vi "Terminate Condition Extract Time.vi"(8 "error in":errorcluster, 11 "Normalized Timer Array in":dbl[][](array[numeric])) -> (0 "error out":errorcluster, 3 "Condition (b) Equilibrium?":bool)   [LabVIEW 2023]
panel:
  out "Numeric":i32
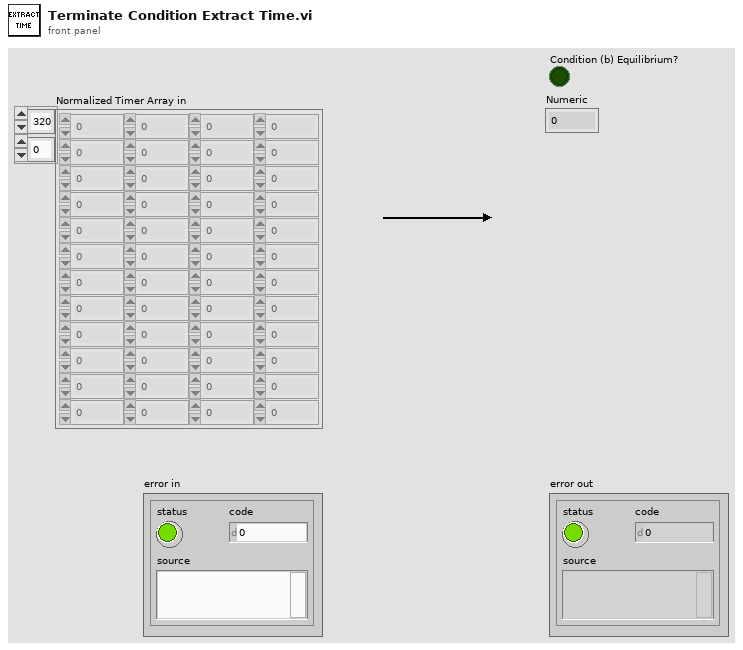
[diagram p1: front panel]
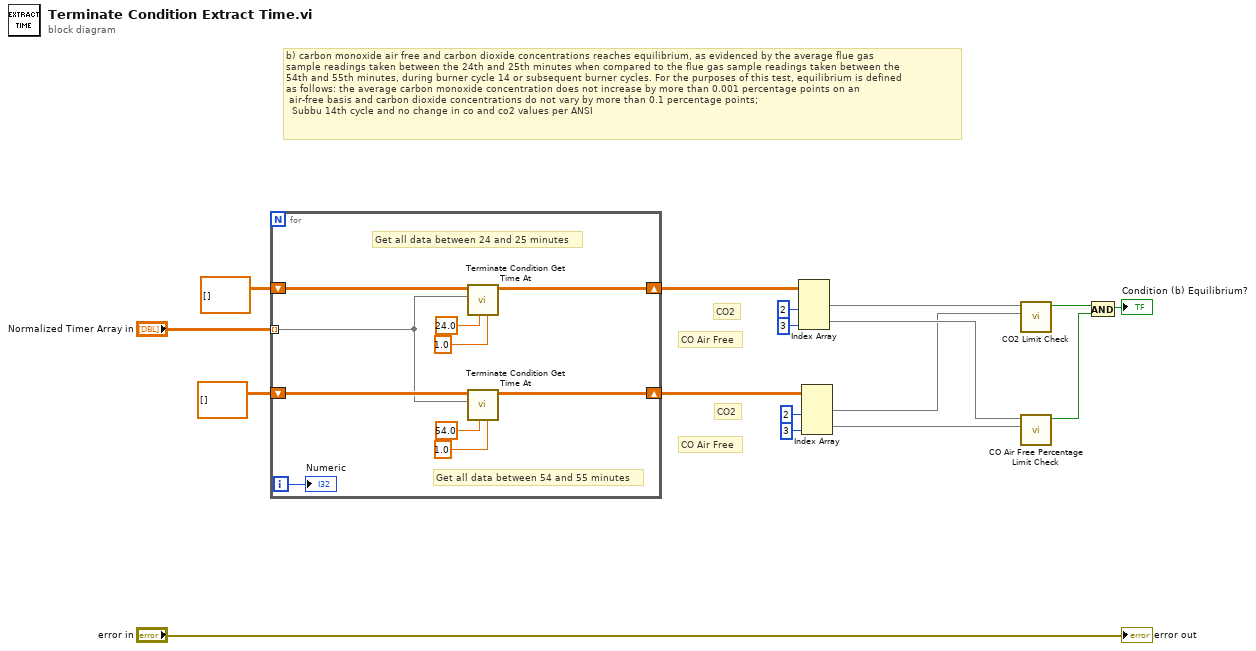
[diagram p0: block diagram]
diagram:
  # "CO Air Free"
  # "CO Air Free"
  # "CO2"
  # "CO2"
  # "b) carbon monoxide air free and carbon dioxide concentrations reaches equilibrium, as evidenced by the average flue gas\nsample readings taken between the 24th and 25th minutes when compared to the flue gas sample readings taken between the\n54th and 55th minutes, during burner cycle 14 or subsequent burner cycles. For the purposes of this test, equilibrium is defined\nas follows: the average carbon monoxide concentration does not increase by more than 0.001 percentage points on an\n air-free basis and carbon dioxide concentrations do not vary by more than 0.1 percentage points;\n  Subbu 14th cycle and no change in co and co2 values per ANSI"
  n1 = for {
    tunnel: "Normalized Timer Array in" -> [w21] mode=indexing
    shift-right: [w26] -> w14
    shift-left: dbl[][] [] -> [w27]
    shift-right: [w22] -> w5
    shift-left: dbl[][] [] -> [w23]
    i -> [w20]
    # "Get all data between 54 and 55 minutes"
    # "Get all data between 24 and 25 minutes"
    n2 = call "Terminate Condition Get Time At.vi"("Minute Adder"=1.0, "Get Time At (Min)"=24.0, "Normalized Timer Array in"=w21, "Array in"=w27) -> ("Array out"=w26:dbl[][])  [unwired: 6 in, 1 out]
    n3 = call "Terminate Condition Get Time At.vi"("Minute Adder"=1.0, "Get Time At (Min)"=54.0, "Normalized Timer Array in"=w21, "Array in"=w23) -> ("Array out"=w22:dbl[][])  [unwired: 6 in, 1 out]
    "Numeric" <- w20
  }
  n4 = Index Array(array=w14, index (col) #1=2 ("disabled index (col)"), index (col) #2=3 ("index (col)")) -> (element #1=w11:dbl[], element #2=w10:dbl[])  [unwired: 2 in]
  n5 = Index Array(array=w5, index (col) #1=2 ("disabled index (col)"), index (col) #2=3 ("index (col)")) -> (element #1=w8:dbl[], element #2=w9:dbl[])  [unwired: 2 in]
  n6 = call "CO2 Limit Check.vi"("54-55 Minutes (CO2)"=w8, "24-25 Minutes (CO2)"=w11) -> ("CO2 In Spec"=w3:bool)  [unwired: 9 in]
  n7 = call "CO Air Free Percentage Limit Check.vi"("54-55 Minutes CO Air Free"=w9, "24-25 Minutes CO Air Free"=w10) -> ("CO Air Free In Spec"=w2:bool)  [unwired: 9 in]
  n8 = And(x=w3, y=w2) -> (x .and. y?=→"Condition (b) Equilibrium?":bool)
  "error out" <- "error in"
